vi "DRIVE_STRAIGHT.vi"(10 "argv":string[](array[string]), 11 "args":u8) -> ()   [LabVIEW 2014]
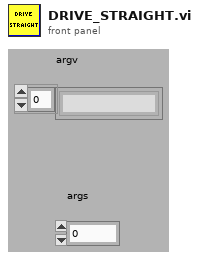
[diagram p1: front panel]
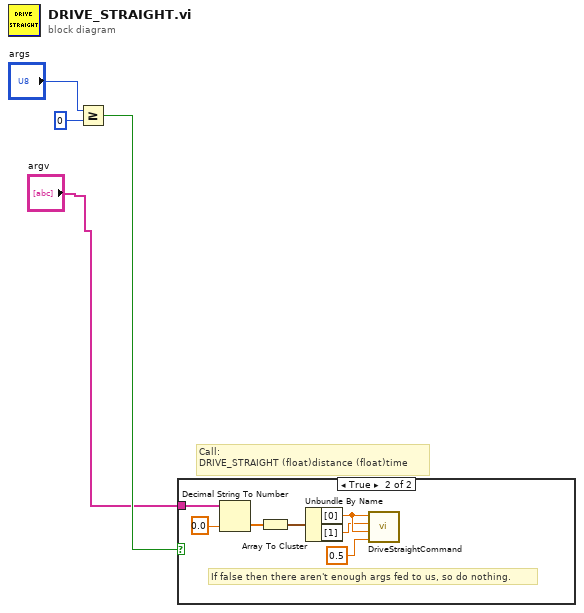
[diagram p0: block diagram]
diagram:
  # "Call:\nDRIVE_STRAIGHT (float)distance (float)time"
  n1 = Greater Or Equal?(x="args", y=u8 0) -> (x >= y?=w4:bool)
  n2 = case shown="True" w4 {
    tunnel: "argv" -> [_ w11]
    frame False {
    }
    frame True {
      # "If false then there aren't enough args fed to us, so do nothing."
      n3 = Decimal String To Number(string=w11, default (0L)=0.0 ("default (0 I32)")) -> (number=w9:dbl[])  [unwired: 2 out]
      n4 = Array To Cluster(array=w9) -> (cluster=w8:cluster{"[0]":dbl, "[1]":dbl})
      n5 = Unbundle By Name(w8) -> ("[0]"=w7:dbl, "[1]"=w6:dbl)
      n6 = call "DriveStraightCommand.vi"("speed"=0.5, "Fwd Bwd"=w7, "Delay ms"=w6, "distance"=w7) -> ()  [unwired: 8 in]
    }
  }
